vi "MessageQueue_Example.vi"() -> ()   [LabVIEW 2016]
doc: "Zeigt die Möglichkeiten der Message Queues auf\n\nsige / 4.12.13"
uses:
  private/MessageQueue.MessageTypeDef.ctl
panel:
  out "ValueEditing":i32
  out "NoOfElementsInQueue":i32
  out "RemainingElements":T1[](array[typedef])
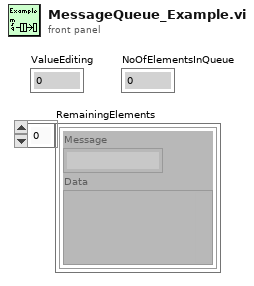
[diagram p1: front panel]
types:
  T1 = typedef "MessageQueue.MessageTypeDef.ctl" = cluster{"Message":string, "Data":variant}
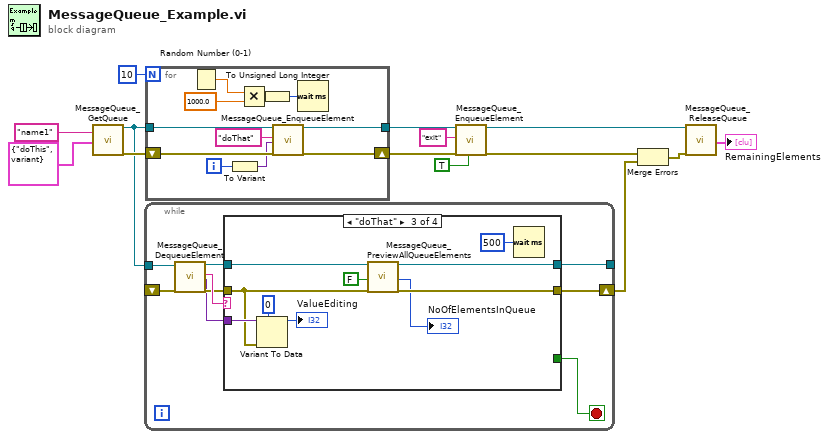
[diagram p0: block diagram]
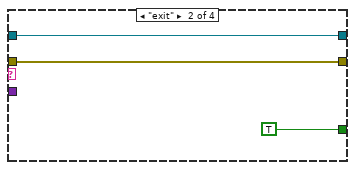
[diagram p3: hidden frame]
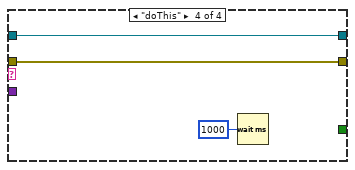
[diagram p4: hidden frame]
diagram:
  n1 = call "MessageQueue_GetQueue.vi"("Name"="name1", "OptionalInitValue"=T1 {"Message"="doThis", "Data"=variant}) -> ("QueueOut"=w6:refnum<queue>, "ErrorOut"=w12:errorcluster)  [unwired: 15 in, 1 out]
  n2 = while {
    tunnel: w6 -> [w23]
    tunnel: [w19] -> _
    shift-right: [w18] -> w2
    shift-left: _ -> [w17]
    stop <- w16 stop-if-true
    n3 = call "MessageQueue_DequeueElement.vi"("QueueIn"=w23, "ErrorIn"=w17) -> ("QueueOut"=w22:refnum<queue>, "Message"=w21:string, "Data"=w15:variant, "ErrorOut"=w20:errorcluster)  [unwired: 13 in, 1 out]
    n4 = case shown="\"doThat\"" w21 {
      tunnel: w22 -> [w24 w27 w33 w39]
      tunnel: w20 -> [w25 w28 w30 w40]
      tunnel: [w24 w27 w38 w39] -> w19
      tunnel: [w25 w28 w37 w40] -> w18
      tunnel: [_ TRUE _ _] -> w16
      tunnel: w15 -> [_ _ w32 _]
      frame Default {
      }
      frame "exit" {
      }
      frame "doThat" {
        n5 = Variant To Data(error in=w30, type=0, Variant=w32) -> (data=→"ValueEditing":i32)  [unwired: 1 out]
        n6 = call "MessageQueue_PreviewAllQueueElements.vi"("QueueIn"=w33, "FlushElements"=FALSE, "ErrorIn"=w30) -> ("QueueOut"=w38:refnum<queue>, "NoOfElementsInQueue"=→"NoOfElementsInQueue":i32, "ErrorOut"=w37:errorcluster)  [unwired: 13 in, 1 out]
        n7 = Wait (ms)(milliseconds to wait=u32 500) -> ()  [unwired: 1 out]
      }
      frame "doThis" {
        n8 = Wait (ms)(milliseconds to wait=u32 1000) -> ()  [unwired: 1 out]
      }
    }
  }
  n9 = for {
    N: 10 -> [_]
    tunnel: w6 -> [w52]
    tunnel: [w49] -> w11
    shift-right: [w48] -> w10
    shift-left: w12 -> [w51]
    i -> [w47]
    n10 = Random Number (0-1)() -> (number: 0 to 1=w45:dbl)
    n11 = To Variant(anything=w47) -> (Variant=w46:variant)
    n12 = Multiply(x=w45, y=1000.0) -> (x*y=w43:dbl)
    n13 = To Unsigned Long Integer(number=w43) -> (unsigned 32bit integer=w42:u32)
    n14 = call "MessageQueue_EnqueueElement.vi"("QueueIn"=w52, "Message"="doThat", "Data"=w46, "ErrorIn"=w51) -> ("QueueOut"=w49:refnum<queue>, "ErrorOut"=w48:errorcluster)  [unwired: 14 in]
    n15 = Wait (ms)(milliseconds to wait=w42) -> ()  [unwired: 1 out]
  }
  n16 = call "MessageQueue_EnqueueElement.vi"("QueueIn"=w11, "Message"="exit", "ErrorIn"=w10, "HighPriority"=TRUE) -> ("QueueOut"=w5:refnum<queue>, "ErrorOut"=w4:errorcluster)  [unwired: 14 in]
  n17 = Merge Errors(w4, w2) -> (w1:errorcluster)
  n18 = call "MessageQueue_ReleaseQueue.vi"("QueueIn"=w5, "ErrorIn"=w1) -> ("RemainingElements"=→"RemainingElements":T1[])  [unwired: 15 in, 2 out]
